vi "set_top_level_VI_ref.vi"(8 "error in (no error)":errorcluster, 10 "top-level VI ref":refnum<vi>, 11 "GenericPlugin.lvclass in":refnum<class "GenericComponent.lvclass">) -> (0 "error out":errorcluster, 3 "GenericPlugin.lvclass out":refnum<class "GenericComponent.lvclass">)   [LabVIEW 2010, in "GenericComponent.lvclass"]
uses:
  GenericComponent.lvclass
  GenericComponent.lvclass/GenericComponent.ctl
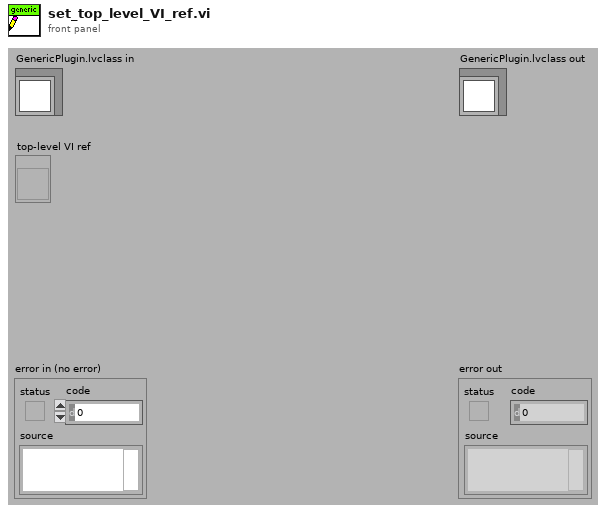
[diagram p1: front panel]
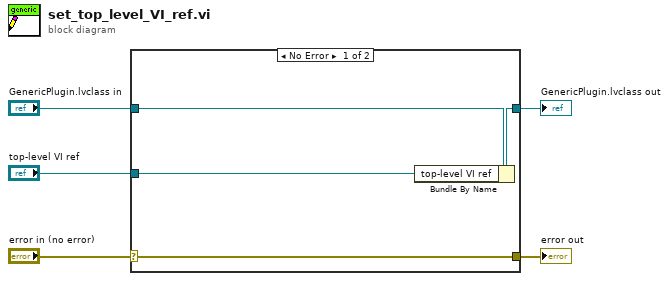
[diagram p0: block diagram]
diagram:
  n1 = case shown="No Error" "error in (no error)" {
    selector: "error in (no error)" -> [w9 w10]
    tunnel: [w9 w10] -> w4
    tunnel: [w7 w11] -> w2
    tunnel: "GenericPlugin.lvclass in" -> [w8 w11]
    tunnel: "top-level VI ref" -> [w6 _]
    frame No Error {
      n2 = Bundle By Name(cluster=w8, "top-level VI ref"=w6) -> (w7:refnum<class "GenericComponent.lvclass">)
    }
    frame Error {
    }
  }
  "error out" <- w4
  "GenericPlugin.lvclass out" <- w2
